vi "obtainOldLibraryPath.vi"(8 "error in (no error)":errorcluster, 11 "Project in":refnum<class "Project.lvclass">) -> (0 "error out":errorcluster, 2 "OldLibPath":path, 3 "Project out":refnum<class "Project.lvclass">)   [LabVIEW 2016, in "Project.lvclass"]
uses:
  Project.lvclass
  Project.lvclass/Project.ctl
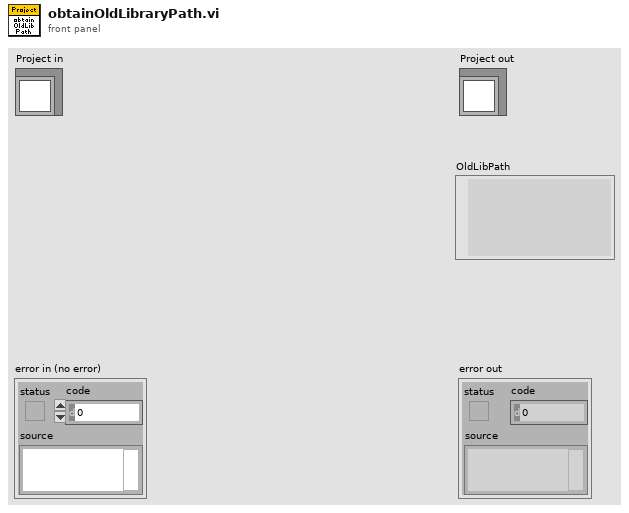
[diagram p1: front panel]
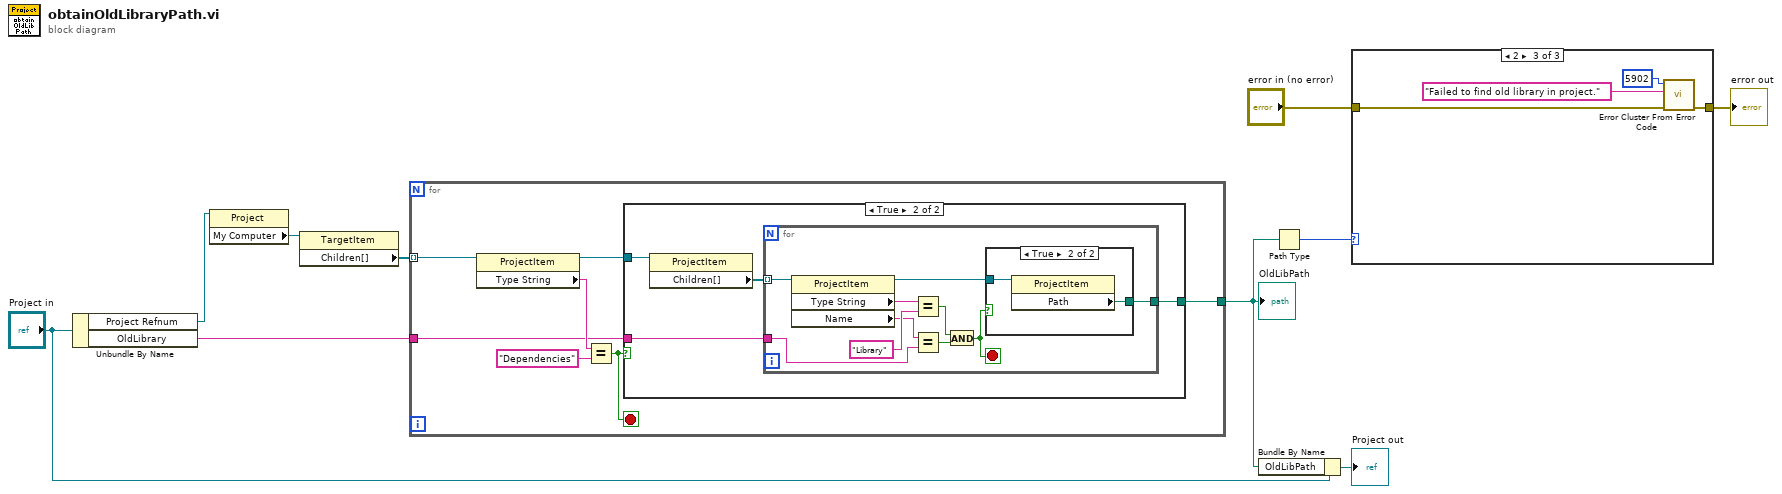
[diagram p0: block diagram]
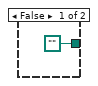
[diagram p4: hidden frame]
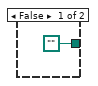
[diagram p5: hidden frame]
diagram:
  n1 = Unbundle By Name("Project in") -> ("Project Refnum"=w8:refnum<vi>, "OldLibrary"=w7:string)
  n2 = property class="Project"(reference=w8) -> ("My Computer"=w10:refnum<vi>)  [unwired: 1 in, 2 out]
  n3 = property class="TargetItem"(reference=w10) -> ("Children[]"=w9:refnum<vi>[])  [unwired: 1 in, 2 out]
  n4 = for {
    tunnel: w9 -> [w17] mode=indexing
    tunnel: w7 -> [w13]
    tunnel: [w12] -> w2
    stop <- w11 stop-if-true
    n5 = property class="ProjectItem"(reference=w17) -> (reference out=w14:refnum<vi>, "Type String"=w16:string)  [unwired: 1 in, 1 out]
    n6 = Equal?(x=w16, y="Dependencies") -> (x = y?=w11:bool)
    n7 = case shown="True" w11 {
      tunnel: w14 -> [_ w22]
      tunnel: w13 -> [_ w20]
      tunnel: [path "" w19] -> w12
      frame False {
      }
      frame True {
        n8 = property class="ProjectItem"(reference=w22) -> ("Children[]"=w21:refnum<vi>[])  [unwired: 1 in, 2 out]
        n9 = for {
          tunnel: w21 -> [w32] mode=indexing
          tunnel: w20 -> [w28]
          tunnel: [w24] -> w19
          stop <- w23 stop-if-true
          n10 = property class="ProjectItem"(reference=w32) -> (reference out=w25:refnum<vi>, "Type String"=w31:string, "Name"=w29:string)  [unwired: 1 in, 1 out]
          n11 = Equal?(x=w31, y="Library") -> (x = y?=w26:bool)
          n12 = Equal?(x=w29, y=w28) -> (x = y?=w27:bool)
          n13 = And(x=w26, y=w27) -> (x .and. y?=w23:bool)
          n14 = case shown="True" w23 {
            tunnel: w25 -> [_ w35]
            tunnel: [path "" w34] -> w24
            frame False {
            }
            frame True {
              n15 = property class="ProjectItem"(reference=w35) -> ("Path"=w34:path)  [unwired: 1 in, 2 out]
            }
          }
        }
      }
    }
  }
  "OldLibPath" <- w2
  n16 = Bundle By Name(cluster="Project in", "OldLibPath"=w2) -> (→"Project out":refnum<class "Project.lvclass">)
  n17 = Path Type(1:w2) -> (0:w6:i16)
  n18 = case shown="2" w6 {
    tunnel: "error in (no error)" -> [w36 w37 w39]
    tunnel: [w36 w37 w38] -> w4
    frame 0, Default {
    }
    frame 1 {
    }
    frame 2 {
      n19 = call <vilib>:"Error Cluster From Error Code.vi"("error in (no error)"=w39, "error message (\"\")"="Failed to find old library in project." ("error message (\"\")"), "error code (0)"=5902) -> ("error out"=w38:errorcluster)  [unwired: 6 in]
    }
  }
  "error out" <- w4
